vi "Lidar2RobotTransform.vi"(0 "z_offset":i16=1000, 1 "y_offset":i16, 2 "x_offset":i16=2000, 5 "Theta_z (deg +/-250)":fxp<+/-,16,9>, 7 "Theta_y (deg +/-250)":fxp<+/-,16,9>, 9 "Angle (deg 0:1:180)":u8, 11 "Range (mm)":u16) -> (6 "X":i16, 8 "Y":i16, 10 "Z":i16)   [LabVIEW 2010]
doc: "Lidar2RobotTransform.vi takes data from the LIDAR and transforms it into cartersian coordinates in the robot's frame of reference.\n\n<b>Inputs</b>\nRange (mm) - range value from LIDAR in mm\nAngle - angle of LIDAR point in integer degrees\nTheta_y - pitch angle of the LIDAR measured degrees below horizontal in range [-250,250]\nTheta_z - yaw of LIDAR measured in degrees left of forwards in range [-250,250]\nx_offset - x offset of LIDAR in robot frame in mm (distance from rear differential to LIDAR)\ny_offset - y offset of LIDAR in robot frame in mm (distance from centerline to LIDAR)\nz_offset - z offset of LIDAR in robot frame in mm (distance from ground to LIDAR)\n\n<b>Outputs</b>\nX - x value of point in robot frame\nY - y value of point in robot frame\nZ - z value of point in robot frame"
panel:
  # "Rear Diff to Mounts (mm)"
  # "Height above Ground (mm)"
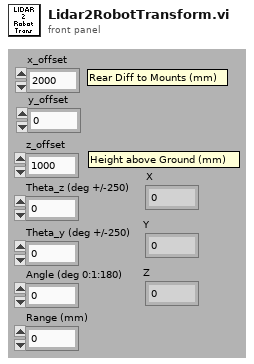
[diagram p1: front panel]
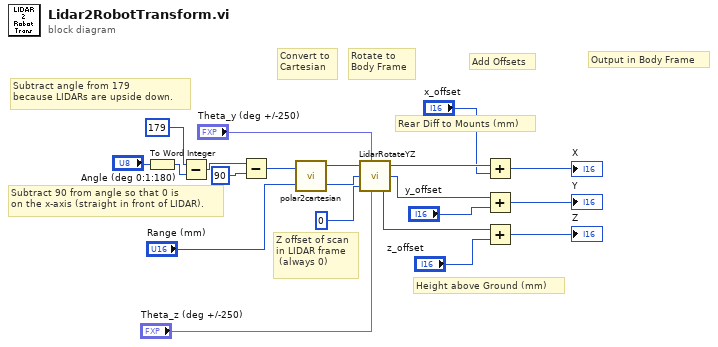
[diagram p0: block diagram]
diagram:
  # "Subtract 90 from angle so that 0 is \non the x-axis (straight in front of LIDAR)."
  # "Subtract angle from 179\nbecause LIDARs are upside down."
  # "Z offset of scan\nin LIDAR frame\n (always 0)"
  # "Height above Ground (mm)"
  # "Rear Diff to Mounts (mm)"
  # "Output in Body Frame"
  # "Add Offsets"
  # "Rotate to\nBody Frame"
  # "Convert to\nCartesian"
  n1 = To Word Integer(number="Angle (deg 0:1:180)") -> (16bit integer=w3:i16)
  n2 = Subtract(x=i16 179 ("y"), y=w3) -> (x-y=w2:i16)
  n3 = Subtract(x=w2, y=i16 90) -> (x-y=w19:i16)
  n4 = call "polar2cartesian.vi"("Range"="Range (mm)", "Angle"=w19) -> ("y"=w16:i16, "x"=w17:i16)
  n5 = call "LidarRotateYZ.vi"("Xin"=w17, "Theta_y (deg +/-250)"="Theta_y (deg +/-250)", "Yin"=w16, "Zin"=i16 0 ("z"), "Theta_z (deg +/-250)"="Theta_z (deg +/-250)") -> ("Xout"=w11:i16, "Yout"=w9:i16, "Zout"=w7:i16)
  n6 = Add(x=w11, y="x_offset") -> (x+y=→"X":i16)
  n7 = Add(x=w9, y="y_offset") -> (x+y=→"Y":i16)
  n8 = Add(x=w7, y="z_offset") -> (x+y=→"Z":i16)
